vi "ClearColumnOf1DArrayCtrl.vi"(10 "차원 크기":i32, 11 "ref array in":refnum<vi>) -> (3 "ref array out":refnum<vi>)   [LabVIEW 2018, in "Library-Ctrl.lvlib"]
uses:
  Library-Ctrl.lvlib
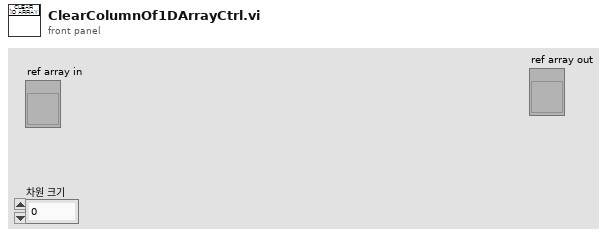
[diagram p1: front panel]
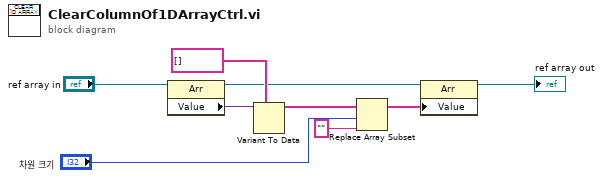
[diagram p0: block diagram]
diagram:
  n1 = property class="Arr"(reference="ref array in") -> (reference out=w4:refnum<vi>, "Value"=w8:variant)  [unwired: 1 in, 1 out]
  n2 = Variant To Data(type=string[] [], Variant=w8) -> (data=w6:string[])  [unwired: 1 in, 1 out]
  n3 = Replace Array Subset(array=w6, new element="", index="차원 크기") -> (w3:string[])
  n4 = property class="Arr"(reference=w4, "Value"=w3) -> (reference out=→"ref array out":refnum<vi>)  [unwired: 1 in, 1 out]
